vi "End by Value.vi"(8 "Error In":errorcluster, 11 "Writer In":refnum<class "Writer.lvclass">) -> (0 "Error Out":errorcluster, 2 "Data":u8[](array[numeric]), 3 "Writer Out":refnum<class "Writer.lvclass">)   [LabVIEW 2018, in "Toolkit.lvlib" / "Writer.lvclass"]
uses:
  Writer.lvclass
  Writer.lvclass/Writer.ctl
  Public/Status/Read Is Error.vi
  Public/Status/Read Status.vi
  Public/Status/Read Status Message.vi
  Public/Data/Read Data Size.vi
  Utility/Status Code.vi
  <vilib>/Utility/error.llb/Error Cluster From Error Code.vi
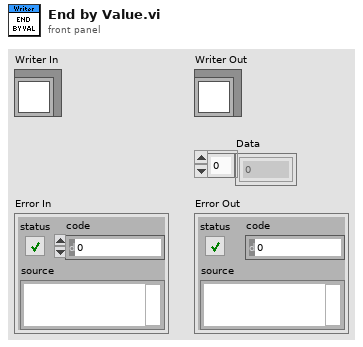
[diagram p1: front panel]
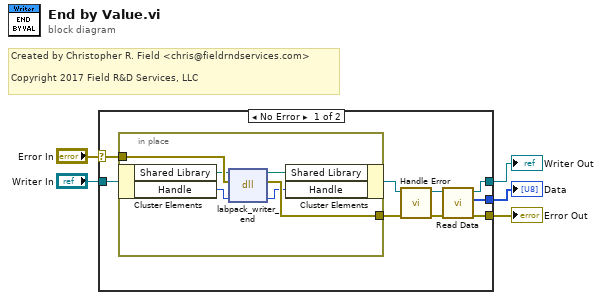
[diagram p0: block diagram]
diagram:
  # "Created by Christopher R. Field <chris@fieldrndservices.com>\n\nCopyright 2017 Field R&D Services, LLC"
  n1 = case shown="No Error" "Error In" {
    selector: "Error In" -> [w14 w22]
    tunnel: [w7 w22] -> w4
    tunnel: "Writer In" -> [w13 w21]
    tunnel: [w9 w21] -> w2
    tunnel: [w6 _] -> w1
    frame No Error {
      n2 = in-place {
        in-place-border: w14 -> [w20]
        in-place-border: [w19] -> w12
        n3 = in-place-cluster #1(w13) -> ("Shared Library"=w18:path, "Handle"=w17:u64)
        n4 = dll-call lib="D:/Users/cfield/Code/MessagePack/LabPack/LabVIEW/trunk/src/LabPack/Private/labpack-x64.dll" fn="labpack_writer_end"(path in=w18, error in=w20, "writer"=w17) -> (path out=w15:path, error out=w19:errorcluster, "writer"=w16:u64)  [unwired: 2 in]
        n5 = in-place-cluster #1("Shared Library"=w15, "Handle"=w16) -> (w11:refnum<class "Writer.lvclass">)
      }
      n6 = call "Handle Error.vi"("Error In"=w12, "Writer In"=w11) -> ("Error Out"=w8:errorcluster, "Writer Out"=w10:refnum<class "Writer.lvclass">)  [unwired: 8 in]
      n7 = call "Read Data.vi"("Error In"=w8, "Writer In"=w10) -> ("Error Out"=w7:errorcluster, "Value"=w6:u8[], "Writer Out"=w9:refnum<class "Writer.lvclass">)  [unwired: 7 in]
    }
    frame Error {
    }
  }
  "Error Out" <- w4
  "Writer Out" <- w2
  "Data" <- w1
